vi "Start Async.vi"(8 "error in (no error)":errorcluster, 11 "gRPC Server in":refnum<class "ServiceName.lvclass">) -> (0 "error out":errorcluster, 3 "gRPC Server out":refnum<class "ServiceName.lvclass">)   [LabVIEW 2019, in "Service Template.lvlib" / "ServiceName.lvclass"]
uses:
  ServiceName.lvclass
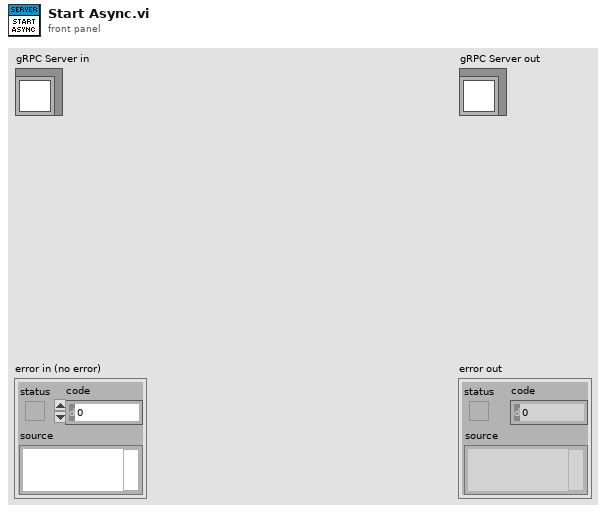
[diagram p1: front panel]
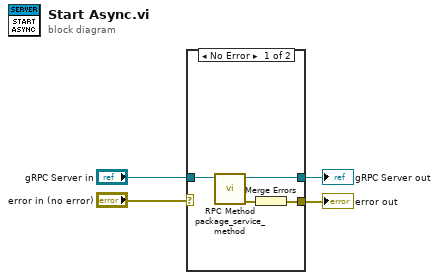
[diagram p0: block diagram]
diagram:
  n1 = case shown="No Error" "error in (no error)" {
    selector: "error in (no error)" -> [_ w10]
    tunnel: [w7 w10] -> w3
    tunnel: [w5 w9] -> w1
    tunnel: "gRPC Server in" -> [w8 w9]
    frame No Error {
      n2 = call "RPC Method package_service_method.vi"("OOP Server in"=w8) -> ("error out"=w6:errorcluster, "OOP Server out"=w5:refnum<class "ServiceName.lvclass">)  [unwired: 9 in]
      n3 = Merge Errors(w6) -> (w7:errorcluster)
    }
    frame Error {
    }
  }
  "error out" <- w3
  "gRPC Server out" <- w1
